vi "Get Build Steps core.vi"(8 "error in (no error)":errorcluster, 9 "Preview?":bool, 10 "Build Configuration":string, 11 "Build Package Item in":refnum<class "Build Package Item.lvclass">) -> (0 "error out":errorcluster, 2 "Build Steps":refnum<class "Build Step.lvclass">[](array[class]))   [LabVIEW 2019, in "VIPM.lvlib" / "Build Package Item.lvclass"]
uses:
  Build Package Item.lvclass
  libs/Solution.lvlibp/Solution/Build Item/Build Step.lvclass
  Build Package Item.lvclass/Build Package Item.ctl
  Open VIPM Step/Open VIPM Step.lvclass
  C:/Users/pasca/source/repos/mgi-solution-explorer-extensions/libs/Solution.lvlibp/Solution/Build Item/Build Step.lvclass
  Build Package Step/Build Package Step.lvclass
  Close VIPM Step/Close VIPM Step.lvclass
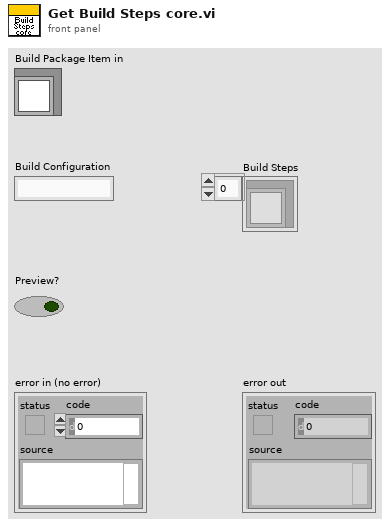
[diagram p1: front panel]
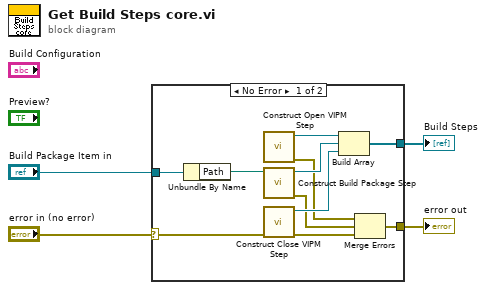
[diagram p0: block diagram]
diagram:
  n1 = case shown="No Error" "error in (no error)" {
    selector: "error in (no error)" -> [w8 w16]
    tunnel: [w15 _] -> w4
    tunnel: [w10 w16] -> w2
    tunnel: "Build Package Item in" -> [w13 _]
    frame No Error {
      n2 = Unbundle By Name(w13) -> ("Path"=w12:path)
      n3 = call "Construct Open VIPM Step.vi"() -> ("error out"=w5:errorcluster, "Open VIPM Step"=w11:refnum<class "Open VIPM Step.lvclass">)  [unwired: 10 in]
      n4 = call "Construct Build Package Step.vi"("Path"=w12) -> ("error out"=w6:errorcluster, "Build Package Step"=w14:refnum<class "Build Package Step.lvclass">)  [unwired: 9 in]
      n5 = call "Construct Close VIPM Step.vi"("error in (no error)"=w8) -> ("error out"=w7:errorcluster, "Close VIPM Step"=w9:refnum<class "Close VIPM Step.lvclass">)  [unwired: 9 in]
      n6 = Build Array(w11, w14, w9) -> (w15:refnum<class "Build Step.lvclass">[])
      n7 = Merge Errors(w5, w6, w7) -> (w10:errorcluster)
    }
    frame Error {
    }
  }
  "error out" <- w2
  "Build Steps" <- w4
